vi "Autonomous Independent.vi"   [LabVIEW 2011]
doc: "This VI is called when autonomous begins, and will automatically be terminated when autonomous ends. You can carry out timed or sensor driven robot movement independently without needing to return to the caller."
uses:
  Robot Global Data.vi
  <vilib>/Rock Robotics/WPI/RobotDrive/WPI_RobotDriveArcadeDrive_Standard(NoSaturation).vi
types:
  T1 = typedef "WPI_JoystickDevRef.ctl" = cluster{"Device":T2}
  T2 = typedef "WPI_JoystickDeviceEnum.ctl" = enum16{"USB 1", "USB 2", "USB 3", "USB 4", "Kinect 1", "Kinect 2"}
  T3 = cluster{"axis 1 (x)":dbl, "axis 2 (y)":dbl, "axis 3 (throttle)":dbl, "axis 4":dbl, "axis 5":dbl, "axis 6":dbl}
  T4 = typedef "WPI_EncoderDevRef.ctl" = cluster{"DevStatus":errorcluster, "EncoderIndex":T5, "CounterIndex":T6, "DistancePerCount":dbl, "Decoding Type":T7}
  T5 = typedef "FPGA_EncoderIdx.ctl" = enum8{"Enc 0", "Enc 1", "Enc 2", "Enc 3", "Invalid"}
  T6 = typedef "FPGA_CounterCtrSystemIndex.ctl" = enum8{"Ctr 0", "Ctr 1", "Ctr 2", "Ctr 3", "Ctr 4", "Ctr 5", "Ctr 6", "Ctr 7", "Invalid"}
  T7 = typedef "WPI_EncoderType.ctl" = enum16{"1x", "2x", "4x"}
  T8 = typedef "WPI_MotorControlDeviceRef.ctl" = cluster{"DeviceStatus":errorcluster, "Type":enum16{"PWM", "CAN"}, "PWM":cluster{"Digital Module":T9, "PWM Channel":T10, "DeadBand":T11}, "CAN":cluster{"Device Number":u8, "Control Mode":T12, "Semaphore":T13, "Max Vout":dbl}, "Invert":bool, "TransformRef":T14, "InvTransformRef":T14}
  T9 = typedef "FPGA_TypedefDigitalModule.ctl" = enum16{"Digital Module 1", "Digital Module 2"}
  T10 = typedef "FPGA_DIOPWMChannel.ctl" = enum8{"PWM 1", "PWM 2", "PWM 3", "PWM 4", "PWM 5", "PWM 6", "PWM 7", "PWM 8", "PWM 9", "PWM 10", "Invalid"}
  T11 = typedef "WPI_PWMDeadband.ctl" = cluster{"Name":string, "maxPositivePwm":i32, "minPositivePwm":i32, "centerPwm":i32, "maxNegativePwm":i32, "minNegativePwm":i32, "angularRange":u16}
  T12 = typedef "WPI_CANJaguar_ControlMode.ctl" = enum8{"Percent VBus", "Current", "Speed", "Position", "Voltage"}
  T13 = typedef "Semaphore RefNum" = refnum<k1>
  T14 = typedef "WPI_PWMTransform_ConPane.ctl" = refnum<vi>
  T15 = typedef "WPI_RobotDriveDevRef.ctl" = cluster{"DevStatus":errorcluster, "Motors[]":T8[], "Square Inputs":bool, "Max Output":dbl, "Isochronous":bool}
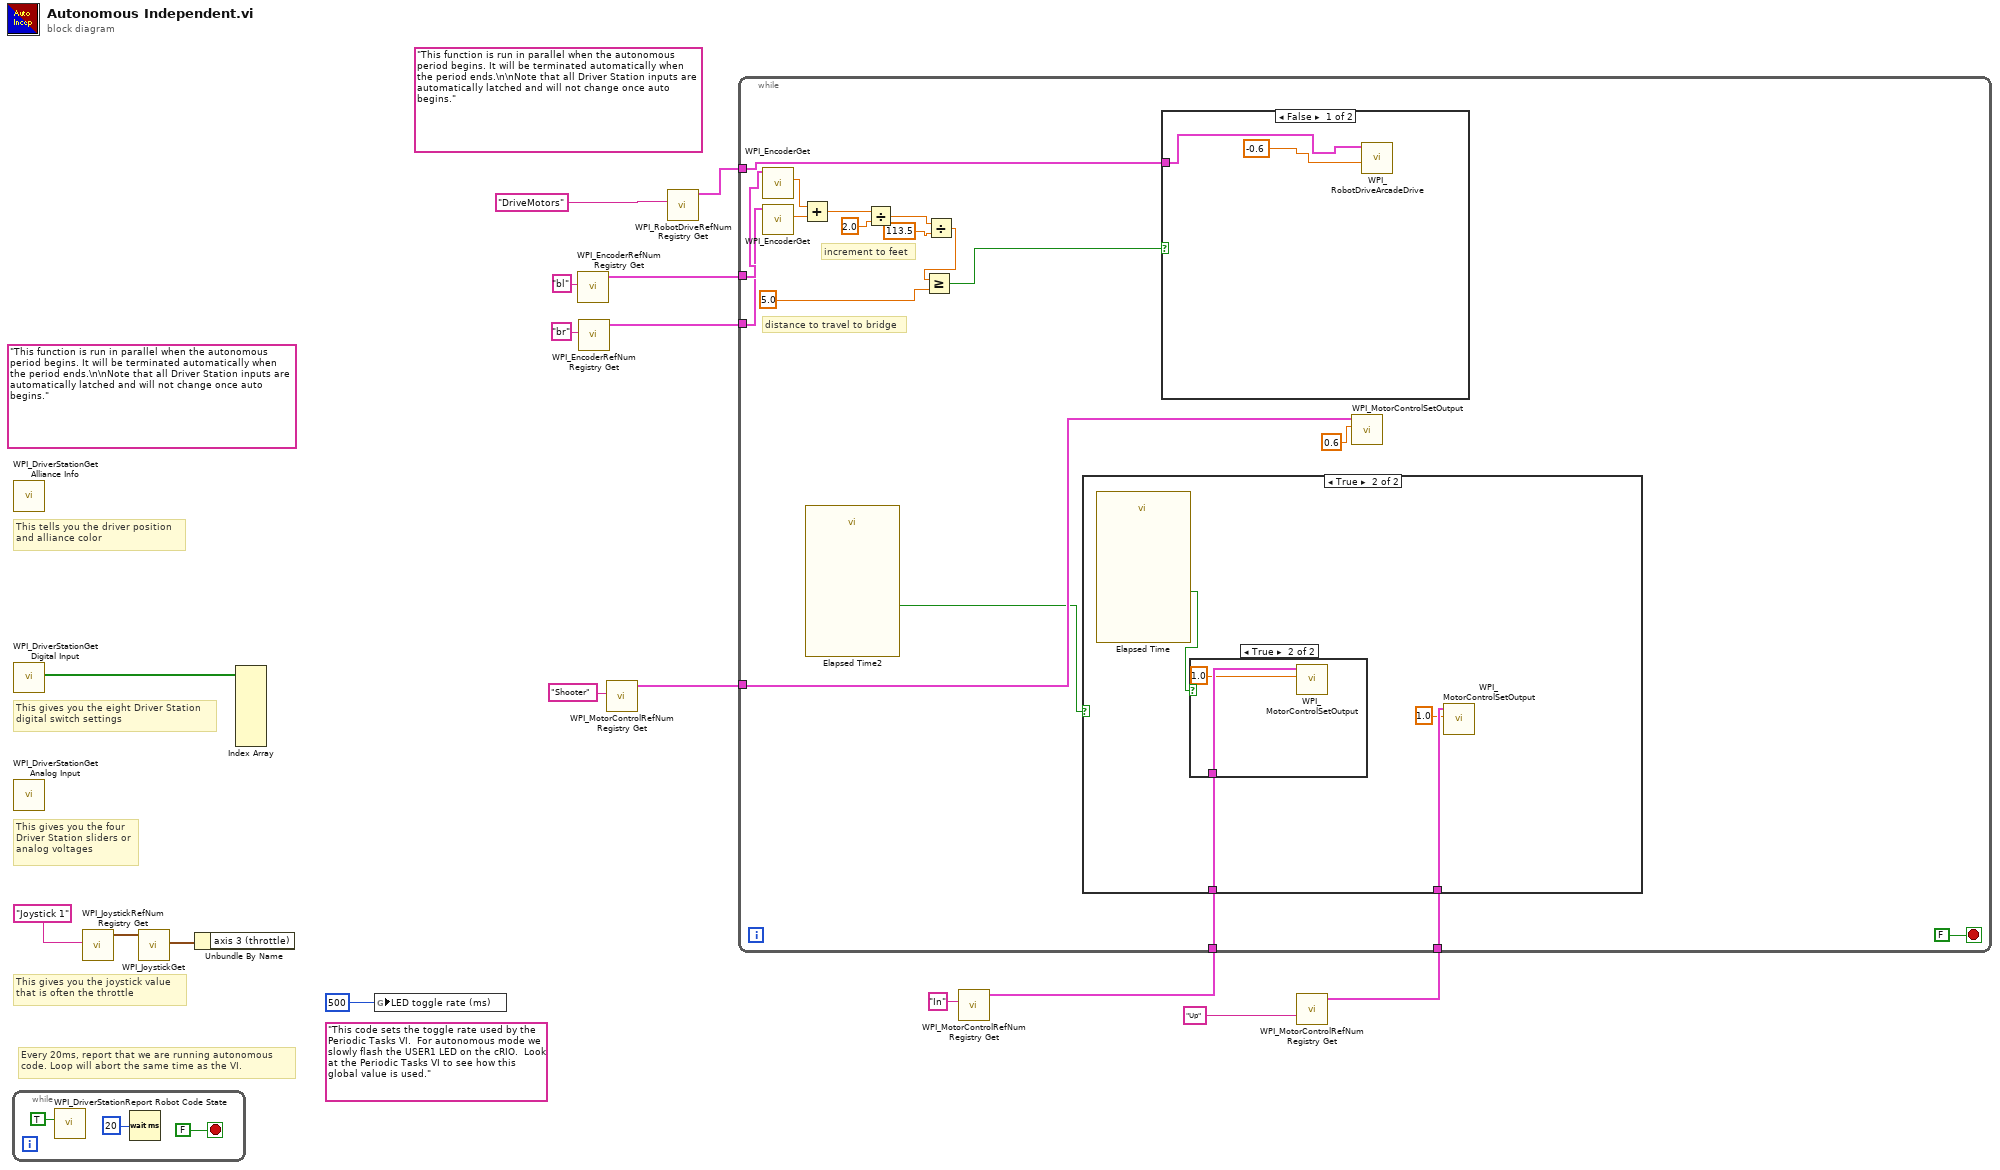
[diagram p0: block diagram]
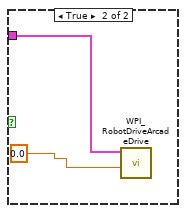
[diagram p2: hidden frame]
diagram:
  (unwired) "This function is run in parallel when the autonomous period begins. It will be terminated automatically when the period ends.\n\nNote that all Driver Station inputs are automatically latched and will not change once auto begins."
  (unwired) "This code sets the toggle rate used by the Periodic Tasks VI.  For autonomous mode we slowly flash the USER1 LED on the cRIO.  Look at the Periodic Tasks VI to see how this global value is used."
  (unwired) "This function is run in parallel when the autonomous period begins. It will be terminated automatically when the period ends.\n\nNote that all Driver Station inputs are automatically latched and will not change once auto begins."
  # "Every 20ms, report that we are running autonomous\ncode. Loop will abort the same time as the VI."
  # "This gives you the joystick value\nthat is often the throttle"
  # "This tells you the driver position\nand alliance color"
  # "This gives you the eight Driver Station\ndigital switch settings"
  # "This gives you the four\nDriver Station sliders or\nanalog voltages"
  n1 = while {
    stop <- FALSE stop-if-true
    n2 = call <vilib>:"WPI_DriverStationReport Robot Code State.vi"("Autonomous"=TRUE) -> ()  [unwired: 10 in, 1 out]
    n3 = Wait (ms)(milliseconds to wait=u32 20) -> ()  [unwired: 1 out]
  }
  n4 = call <vilib>:"WPI_DriverStationGet Alliance Info.vi"() -> ()  [unwired: 12 out]
  n5 = call <vilib>:"WPI_DriverStationGet Digital Input.vi"() -> ("Driver Station Digital Input (1-8)"=w17:bool[])  [unwired: 11 out]
  n6 = call <vilib>:"WPI_DriverStationGet Analog Input.vi"() -> ()  [unwired: 12 out]
  n7 = call <vilib>:"WPI_JoystickRefNum Registry Get.vi"("refnum name"="Joystick 1") -> ("JoystickDevRef"=w14:T1)  [unwired: 1 in, 9 out]
  n8 = call <vilib>:"WPI_JoystickGet.vi"("JoystickDevRef"=w14) -> ("Axes"=w15:T3)  [unwired: 1 in, 5 out]
  n9 = Unbundle By Name(w15) -> ()  [unwired: 1 out]
  n10 = Index Array(array=w17) -> ()  [unwired: 8 in, 8 out]
  n11 = global write "Robot Global Data.vi" "LED toggle rate (ms)"(u32 500 ("LED ms toggle rate")) -> ()
  n12 = call <vilib>:"WPI_EncoderRefNum Registry Get.vi"("refnum name"="bl") -> ("EncoderDevRef"=w12:T4)  [unwired: 9 in, 1 out]
  n13 = call <vilib>:"WPI_EncoderRefNum Registry Get.vi"("refnum name"="br") -> ("EncoderDevRef"=w11:T4)  [unwired: 9 in, 1 out]
  n14 = call <vilib>:"WPI_MotorControlRefNum Registry Get.vi"("refnum name"="Shooter") -> ("MotorControlDevRef"=w2:T8)  [unwired: 9 in, 1 out]
  n15 = call <vilib>:"WPI_RobotDriveRefNum Registry Get.vi"("refnum name"="DriveMotors") -> ("RobotDriveDevRef"=w7:T15)  [unwired: 9 in, 1 out]
  n16 = call <vilib>:"WPI_MotorControlRefNum Registry Get.vi"("refnum name"="In") -> ("MotorControlDevRef"=w5:T8)  [unwired: 9 in, 1 out]
  n17 = call <vilib>:"WPI_MotorControlRefNum Registry Get.vi"("refnum name"="Up") -> ("MotorControlDevRef"=w6:T8)  [unwired: 9 in, 1 out]
  n18 = while {
    tunnel: w12 -> [w38]
    tunnel: w11 -> [w37]
    tunnel: w7 -> [w32]
    tunnel: w6 -> [w31]
    tunnel: w5 -> [w30]
    tunnel: w2 -> [w28]
    stop <- FALSE stop-if-true
    # "increment to feet"
    # "distance to travel to bridge"
    n19 = call <vilib>:"WPI_EncoderGet.vi"("EncoderDevRef"=w38) -> ("Distance"=w36:dbl)  [unwired: 5 in, 5 out]
    n20 = call <vilib>:"WPI_EncoderGet.vi"("EncoderDevRef"=w37) -> ("Distance"=w35:dbl)  [unwired: 5 in, 5 out]
    n21 = Add(x=w36, y=w35) -> (x+y=w34:dbl)
    n22 = call "Elapsed Time2"() -> ("Time has Elapsed"=w21:bool)  [unwired: 12 in, 7 out]
    n23 = Divide(x=w34, y=2.0) -> (x/y=w26:dbl)
    n24 = Divide(x=w26, y=113.5) -> (x/y=w24:dbl)
    n25 = Greater Or Equal?(x=w24, y=5.0) -> (x >= y?=w22:bool)
    n26 = case shown="True" w21 {
      tunnel: w31 -> [_ w46]
      tunnel: w30 -> [_ w45]
      frame False {
      }
      frame True {
        n27 = call "Elapsed Time"() -> ("Time has Elapsed"=w43:bool)  [unwired: 12 in, 7 out]
        n28 = case shown="True" w43 {
          tunnel: w45 -> [_ w48]
          frame False {
          }
          frame True {
            n29 = call <vilib>:"WPI_MotorControlSetOutput.vi"("Output"=1.0, "MotorControlDevRef"=w48) -> ()  [unwired: 8 in, 2 out]
          }
        }
        n30 = call <vilib>:"WPI_MotorControlSetOutput.vi"("Output"=1.0, "MotorControlDevRef"=w46) -> ()  [unwired: 8 in, 2 out]
      }
    }
    n31 = case shown="False" w22 {
      tunnel: w32 -> [w39 w42]
      frame False {
        n32 = call-poly <vilib>:"WPI_RobotDriveArcadeDrive.vi"("Y axis value"=-0.6 ("t"), "RobotDriveDevRef"=w39) -> ()  [unwired: 8 in, 2 out]
      }
      frame True {
        n33 = call-poly <vilib>:"WPI_RobotDriveArcadeDrive.vi"("Y axis value"=0.0 ("t"), "RobotDriveDevRef"=w42) -> ()  [unwired: 8 in, 2 out]
      }
    }
    n34 = call <vilib>:"WPI_MotorControlSetOutput.vi"("Output"=0.6, "MotorControlDevRef"=w28) -> ()  [unwired: 8 in, 2 out]
  }
